vi "Save calibration profile image sequence.vi"(8 "Error In":errorcluster, 10 "Image In":T1[](array[typedef]), 11 "folder path":path) -> (0 "Error Out":errorcluster)   [LabVIEW 2020]
uses:
  <vilib>/vision/Image Controls.llb/IMAQ Image.ctl
  <vilib>/vision/NI_Vision_Development_Module.lvlib
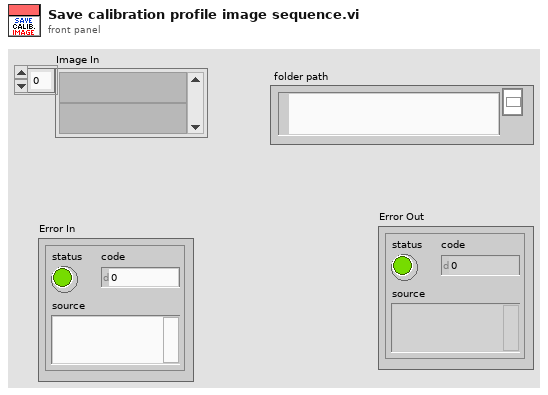
[diagram p1: front panel]
types:
  T1 = typedef "IMAQ Image.ctl" = refnum<image>
  T2 = typedef "Fixed strings.ctl" = cluster{"ROI file name":string, "Normalised ROI file name":string, "Zplane Pockels values file name":string, "Functional data folder name":string, "Experiment Header file name":string, "Z-stack images folder name":string, "Groups setup rel. path":string, "Groups text file rel. path":string, "TDMS files folder name (F.img)":string, "TDMS files folder name (V.acq)":string, "TDMS files folder name (Pl.acq)":string, "Cycle rel times sequence file":string, "Dynamically called VIs folder name":string, "Time Series folder base name":string, "Parameter Sweep":string, "Calibration Profile Images":string}
  T3 = typedef "Image Type" = u32
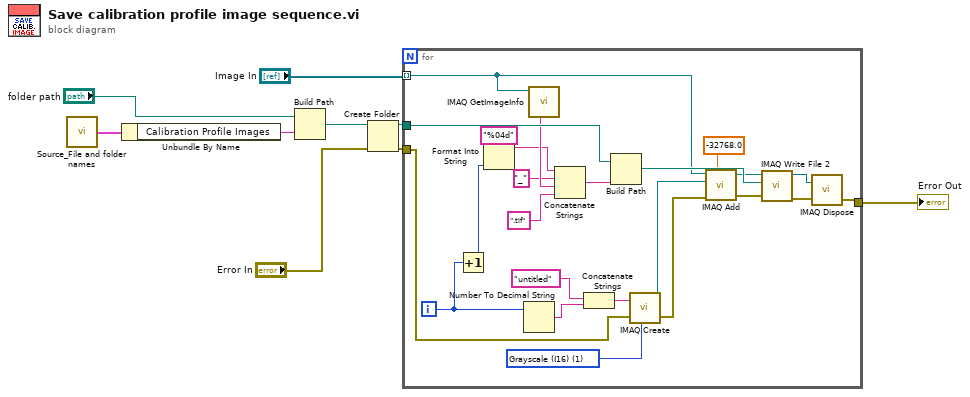
[diagram p0: block diagram]
diagram:
  n1 = call "Source_File and folder names.vi"() -> ("Fixed strings"=w6:T2)  [unwired: 1 in]
  n2 = Unbundle By Name(w6) -> ("Calibration Profile Images"=w7:string)
  n3 = Build Path(base path="folder path", name or relative path=w7) -> (appended path=w3:path)
  n4 = Create Folder(path (use dialog)=w3, error in="Error In") -> (created path=w2:path, error out=w1:errorcluster)  [unwired: 1 in, 1 out]
  n5 = for {
    tunnel: w2 -> [w23]
    tunnel: w1 -> [w22]
    tunnel: [w24] -> w9
    tunnel: "Image In" -> [w19] mode=indexing
    i -> [w11]
    w33 = T3 1 items=["Grayscale (U8)", "Grayscale (I16)", "Grayscale (SGL)", "Complex (CSG)", "RGB (U32)", "HSL (U32)", "RGB (U64)"] ("Image Type")
    n6 = Increment(x=w11) -> (x+1=w10:i32)
    n7 = Format Into String(format string="%04d", w10) -> (resulting string=w13:string)  [unwired: 2 in, 1 out]
    n8 = Number To Decimal String(number=w11) -> (decimal integer string=w28:string)  [unwired: 1 in]
    n9 = call "IMAQ GetImageInfo"("Image"=w19) -> ("Image Name"=w17:string)  [unwired: 3 in, 7 out]
    n10 = Concatenate Strings(w13, "_" ("string"), w17, ".tif" ("string")) -> (w15:string)
    n11 = Concatenate Strings("untitled" ("Image Name"), w28) -> (w27:string)
    n12 = Build Path(base path=w23, name or relative path=w15) -> (appended path=w31:path)
    n13 = call "IMAQ Create"("Image Name"=w27, "Image Type"=w33, "error in (no error)"=w22) -> ("New Image"=w32:T1, "error out"=w21:errorcluster)  [unwired: 2 in]
    n14 = call "IMAQ Add"("Image Src A"=w19, "Constant"=-32768.0, "Image Dst"=w32, "error in (no error)"=w21) -> ("Image Dst Out"=w30:T1, "error out"=w20:errorcluster)  [unwired: 3 in]
    n15 = call-poly "IMAQ Write File 2"("error in (no error)"=w20, "File Path"=w31, "Image"=w30) -> ("error out"=w25:errorcluster, "Image Out (duplicate)"=w26:T1)  [unwired: 7 in]
    n16 = call "IMAQ Dispose"("Image"=w26, "error in (no error)"=w25) -> ("error out"=w24:errorcluster)  [unwired: 4 in]
  }
  "Error Out" <- w9
